vi "event_subscriber2.vi"() -> ()   [LabVIEW 2016]
uses:
  ts_sallv_exa/SALLV_EXA.lvlib
panel:
  out "State":T1(ring)
  out "Heartbean?":bool=TRUE
  out "Count":i32
  out "Stop 2":bool=TRUE
  out "Stop":bool=TRUE
  in  "stop":bool
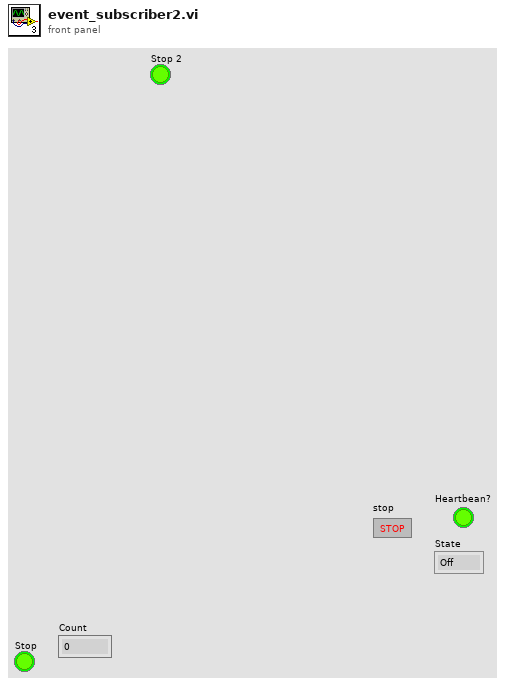
[diagram p1: front panel]
types:
  T1 = enum16{"Off", "Standby", "Enable", "Disable", "Fault"}
  T2 = typedef "SALLV_EXA.lvlib/logevent_Heartbeat.ctl" = cluster{"Heartbeat":bool, "priority":i32}
  T3 = typedef "SALLV_EXA.lvlib/logevent_SummaryState.ctl" = cluster{"SummaryStateValue":i32, "priority":i32}
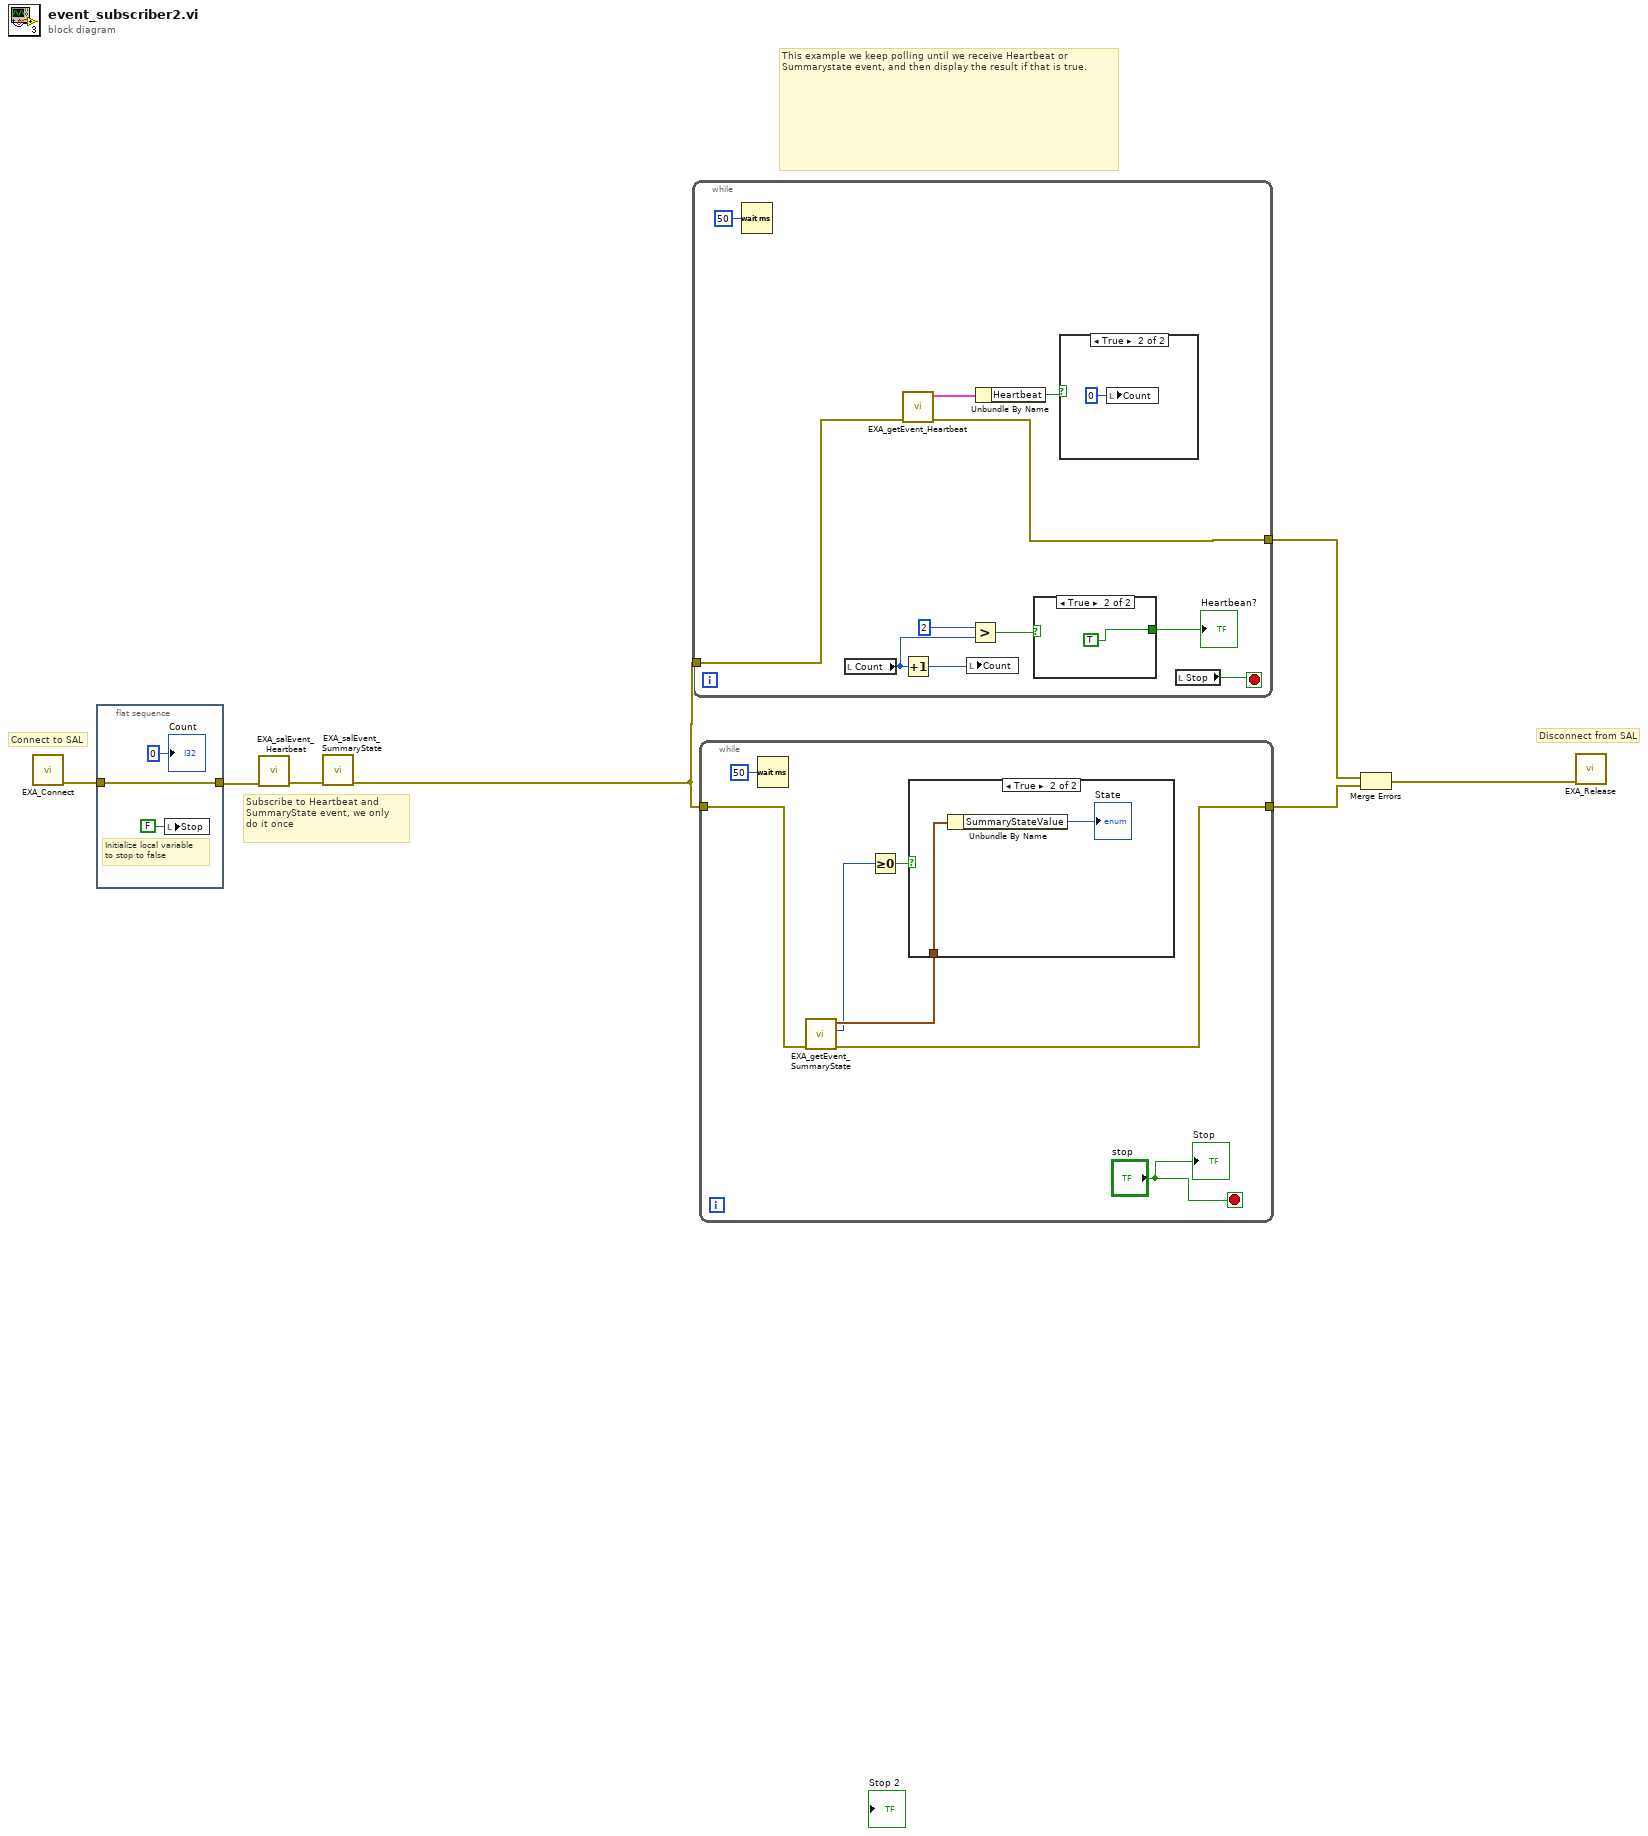
[diagram p0: block diagram]
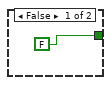
[diagram p3: hidden frame]
diagram:
  # "This example we keep polling until we receive Heartbeat or Summarystate event, and then display the result if that is true."
  # "Subscribe to Heartbeat and SummaryState event, we only\ndo it once"
  # "Disconnect from SAL"
  # "Connect to SAL"
  n1 = call "EXA_Connect.vi"() -> ("error out"=w7:errorcluster)  [unwired: 10 in, 1 out]
  n2 = flat-sequence {
    tunnel: w7 -> [w9]
    tunnel: [w9] -> w4
    frame #0 {
      # "Initialize local variable \nto stop to false"
      n3 = local write "Stop"(FALSE ("Stop")) -> ()
      "Count" <- 0 ("Count")
    }
  }
  n4 = call "EXA_salEvent_Heartbeat.vi"("error in (no error)"=w4) -> ("error out"=w5:errorcluster)  [unwired: 9 in, 1 out]
  n5 = call "EXA_salEvent_SummaryState.vi"("error in (no error)"=w5) -> ("error out"=w3:errorcluster)  [unwired: 9 in, 1 out]
  n6 = while {
    tunnel: w3 -> [w20]
    tunnel: [w19] -> w2
    stop <- w21 stop-if-true
    n7 = Wait (ms)(milliseconds to wait=u32 50) -> ()  [unwired: 1 out]
    n8 = local read "Count"() -> (w14:i32)
    n9 = call "EXA_getEvent_Heartbeat.vi"("error in (no error)"=w20) -> ("error out"=w19:errorcluster, "logevent_Heartbeat_Ctl out"=w13:T2)  [unwired: 8 in, 1 out]
    n10 = Increment(x=w14) -> (x+1=w15:i32)
    n11 = local write "Count"(w15) -> ()
    n12 = Greater?(x=2 ("y"), y=w14) -> (0:w17:bool)
    n13 = Unbundle By Name(w13) -> ("Heartbeat"=w12:bool)
    n14 = case shown="True" w17 {
      tunnel: [FALSE TRUE] -> w18
      frame False {
      }
      frame True {
      }
    }
    "Heartbean?" <- w18
    n15 = case shown="True" w12 {
      frame False {
      }
      frame True {
        n16 = local write "Count"(0 ("Count")) -> ()
      }
    }
    n17 = local read "Stop"() -> (w21:bool)
  }
  n18 = while {
    tunnel: w3 -> [w28]
    tunnel: [w29] -> w6
    stop <- "stop" stop-if-true
    n19 = Wait (ms)(milliseconds to wait=u32 50) -> ()  [unwired: 1 out]
    n20 = call "EXA_getEvent_SummaryState.vi"("error in (no error)"=w28) -> ("error out"=w29:errorcluster, "function return"=w26:i32, "logevent_SummaryState_Ctl out"=w30:T3)  [unwired: 8 in]
    n21 = Greater Or Equal To 0?(x=w26) -> (x >= 0?=w27:bool)
    n22 = case shown="True" w27 {
      tunnel: w30 -> [_ w33]
      frame False {
      }
      frame True {
        n23 = Unbundle By Name(w33) -> ("SummaryStateValue"=→"State":i32)
      }
    }
    "Stop" <- "stop"
  }
  n24 = Merge Errors(w2, w6) -> (w1:errorcluster)
  n25 = call "EXA_Release.vi"("error in (no error)"=w1) -> ()  [unwired: 9 in, 2 out]
